vi "Unpad DetectorInfo.vi"(1 "Detector Info":T2) -> (0 "Detector Info out":T1)   [LabVIEW 2018]
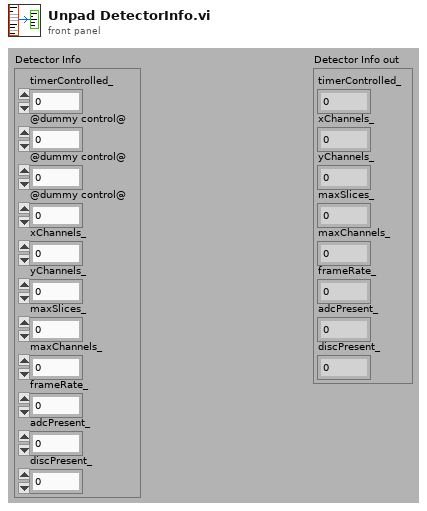
[diagram p1: front panel]
types:
  T1 = cluster{"timerControlled_":u8, "xChannels_":i32, "yChannels_":i32, "maxSlices_":i32, "maxChannels_":i32, "frameRate_":i32, "adcPresent_":u8, "discPresent_":u8}
  T2 = cluster{"timerControlled_":u8, "@dummy control@":i8, "@dummy control@":i8, "@dummy control@":i8, "xChannels_":i32, "yChannels_":i32, "maxSlices_":i32, "maxChannels_":i32, "frameRate_":i32, "adcPresent_":u8, "discPresent_":u8}
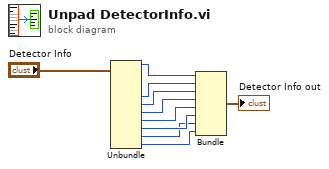
[diagram p0: block diagram]
diagram:
  n1 = Unbundle("Detector Info") -> ("timerControlled_"=w9:u8, "xChannels_"=w8:i32, "yChannels_"=w7:i32, "maxSlices_"=w6:i32, "maxChannels_"=w5:i32, "frameRate_"=w4:i32, "adcPresent_"=w3:u8, "discPresent_"=w2:u8)  [unwired: 3 out]
  n2 = Bundle("timerControlled_"=w9, "xChannels_"=w8, "yChannels_"=w7, "maxSlices_"=w6, "maxChannels_"=w5, "frameRate_"=w4, "adcPresent_"=w3, "discPresent_"=w2) -> (→"Detector Info out":T1)  [unwired: 1 in]
